vi "Cam0 Ball Target Loop.vi"(0 "Camera Name":string="cam0") -> ()   [LabVIEW 2023]
uses:
  <vilib>/vision/Image Controls.llb/IMAQ Image.ctl
  Camera Set Up/Event Setup Types.ctl
  <vilib>/Rock Robotics/Network Tables/NT Write Numeric Array.vi
  <vilib>/Utility/config.llb/Write Key (String).vi
  <vilib>/Utility/config.llb/Read Key (String).vi
  <vilib>/Utility/config.llb/NI_LVConfig.lvlib
  <vilib>/vision/NI_Vision_Development_Module.lvlib
panel:
  in  "Main":enum32{"Page 1", "Page 2"}(tab)
  out "Algae Distance":dbl[](array[numeric]) caption="Distance" format="%.1f"
  out "Algae Angle":dbl[](array[numeric]) caption="Angle" format="%.1f"
  out "Image":T1(plugin-control)
  in  "Settings":bool
  in  "Save":bool
  in  "Tools":bool
  in  "Home":bool
  out "Ball Fps":dbl format="%#.0f"
  in  "Ball Diameter (in)":dbl=16.0
  in  "FOV":dbl=68.5
  in  "Algae Color Range":T2={"Hue"={21.620689392089844, 69.62068939208984}, "Sat"={66.41378784179688, 255.0}, "Val"={96.0, 255.0}} caption="Color Range" {"Hue" scale=0.0..255.0 scale format="%#_3g"}
  out "Mask":T1(plugin-control)
  in  "Score Threshold %":dbl=80.0
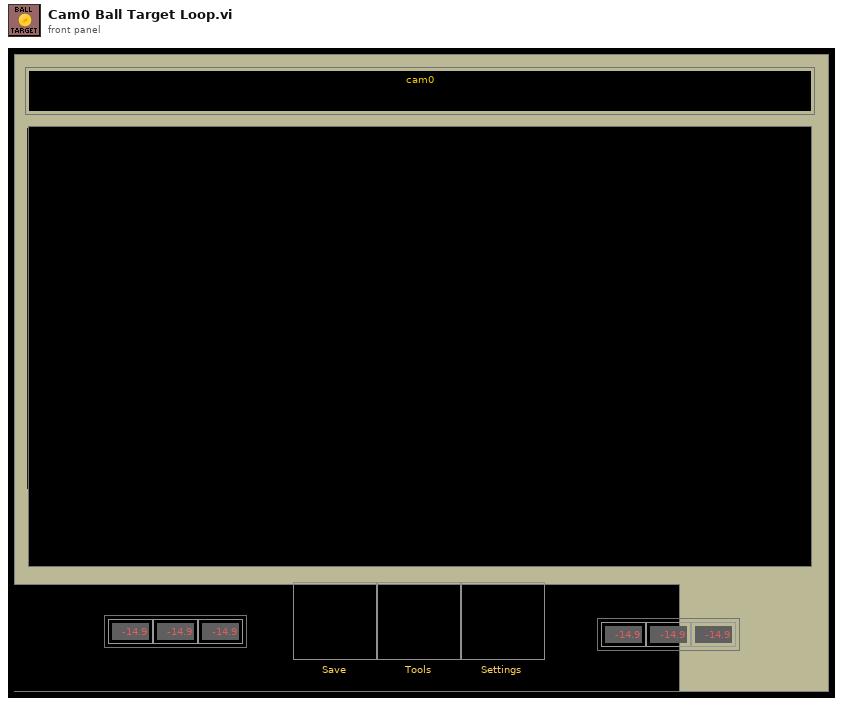
[diagram p1: front panel]
types:
  T1 = typedef "IMAQ Image.ctl" = refnum<image>
  T2 = cluster{"Hue":cluster{dbl, dbl}, "Sat":cluster{dbl, dbl}, "Val":cluster{dbl, dbl}}
  T3 = typedef "Particle Parameters" = i32
  T4 = typedef "Image Type" = u32
  T5 = typedef "Event Setup Types.ctl" = enum16{"Default", "Camera Loop Started", "Save Data", "Open Front Panel", "Exit"}
  T6 = typedef "Target Fields.ctl" = cluster{"diameter points":cluster{"first point":cluster{"x":dbl, "y":dbl}, "projected point":cluster{"x":dbl, "y":dbl}}, "normalized center":cluster{"x":dbl, "y":dbl}, "Overall Score":dbl, "Area Score":dbl, "Moment Score":dbl, "Aspect Score":dbl, "Distance (ft)":dbl, "Upper Goal":bool}
  T7 = typedef "NI_LVConfig.lvlib/Config Data RefNum.ctl" = refnum<k1>
  T8 = cluster{cluster{"Lower":dbl, "Upper":dbl}, cluster{"Lower":dbl, "Upper":dbl}, cluster{"Lower":dbl, "Upper":dbl}}
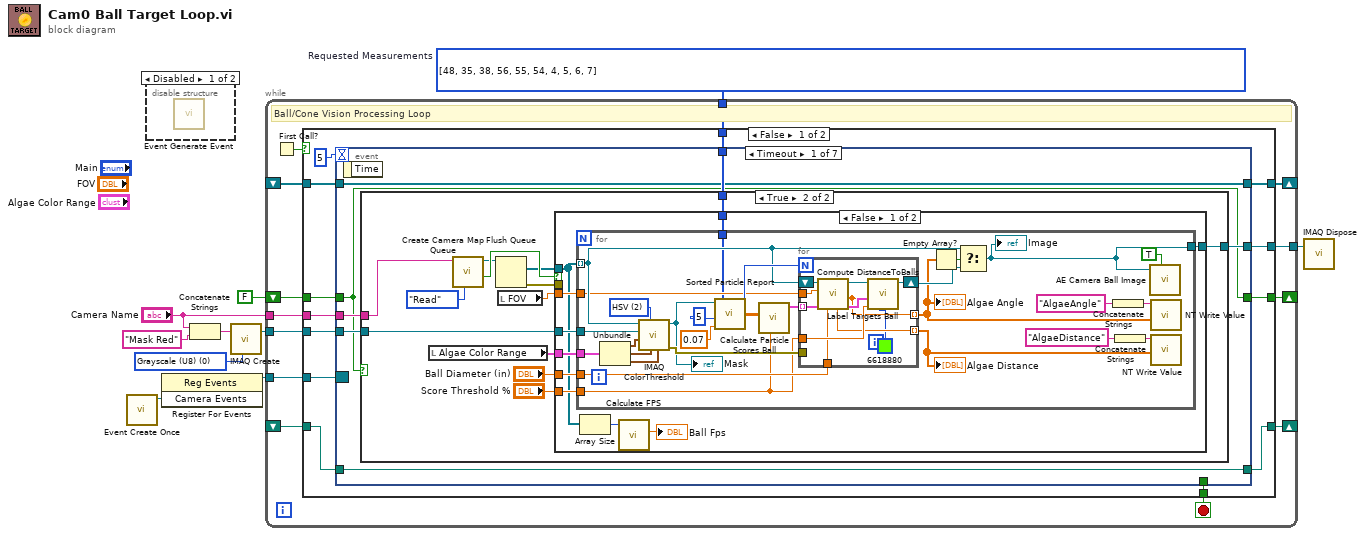
[diagram p0: block diagram]
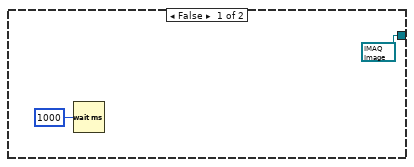
[diagram p3: hidden frame]
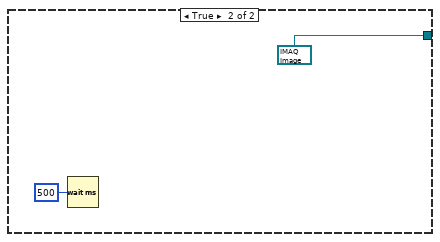
[diagram p4: hidden frame]
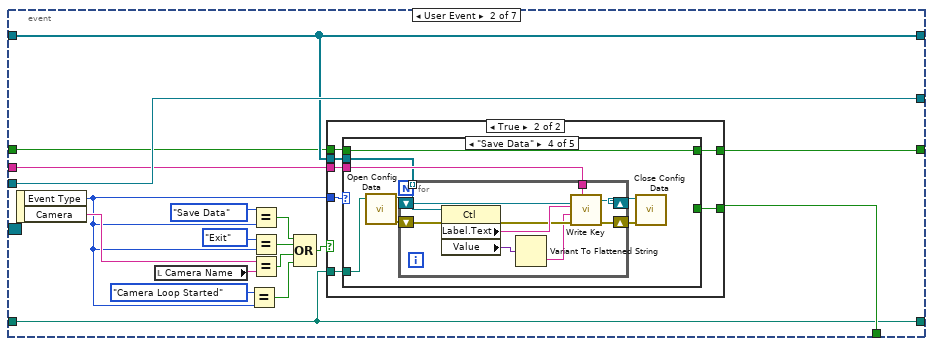
[diagram p5: hidden frame]
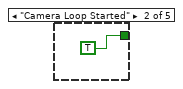
[diagram p8: hidden frame]
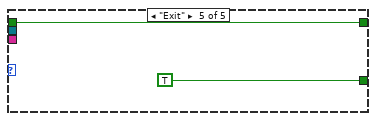
[diagram p10: hidden frame]
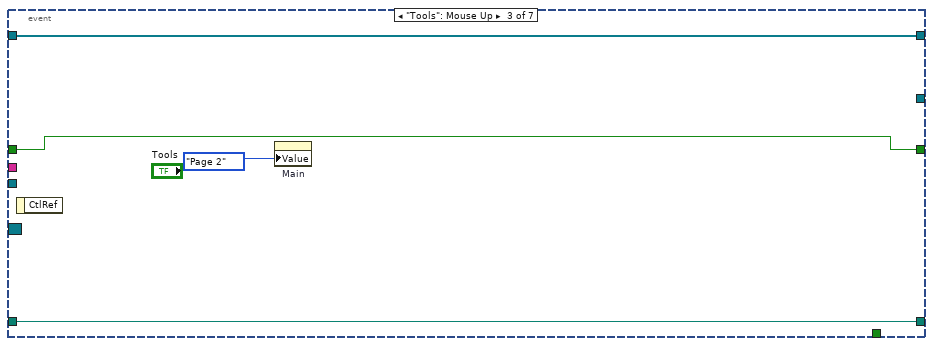
[diagram p11: hidden frame]
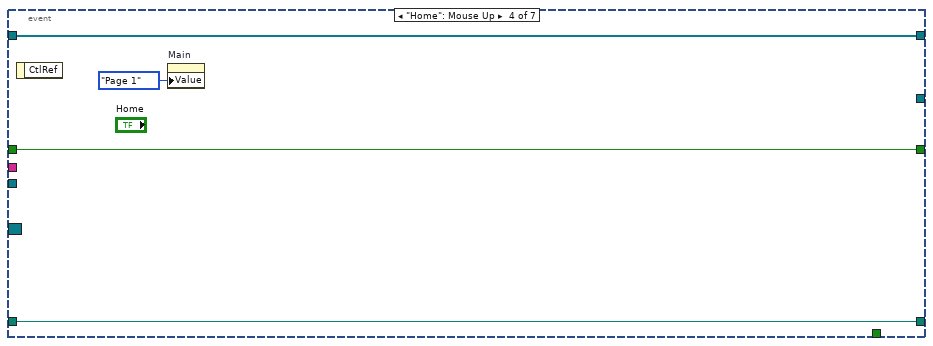
[diagram p12: hidden frame]
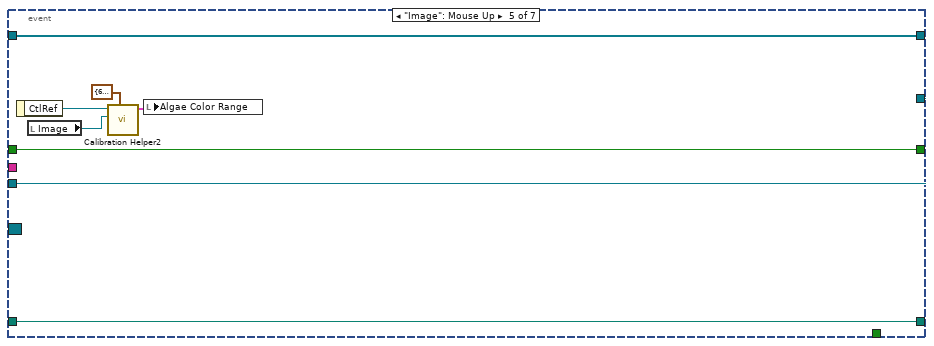
[diagram p13: hidden frame]
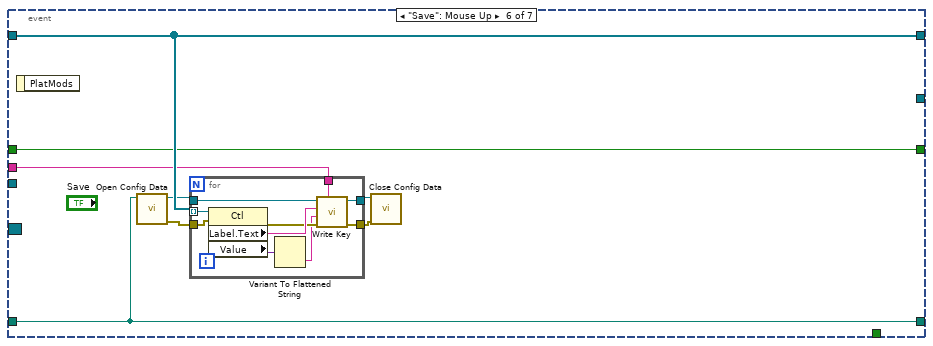
[diagram p14: hidden frame]
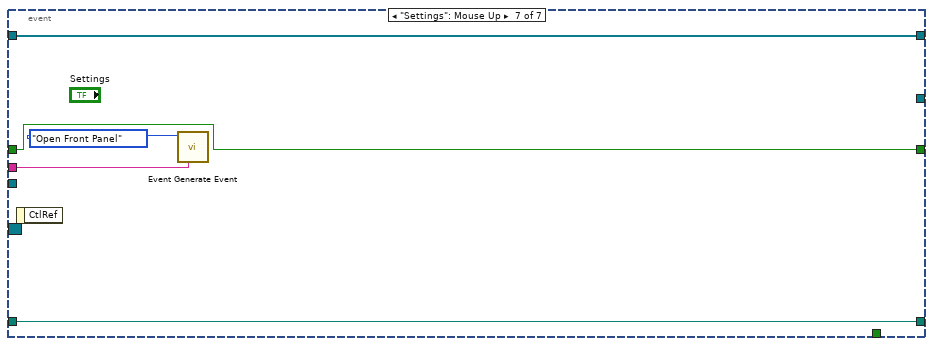
[diagram p15: hidden frame]
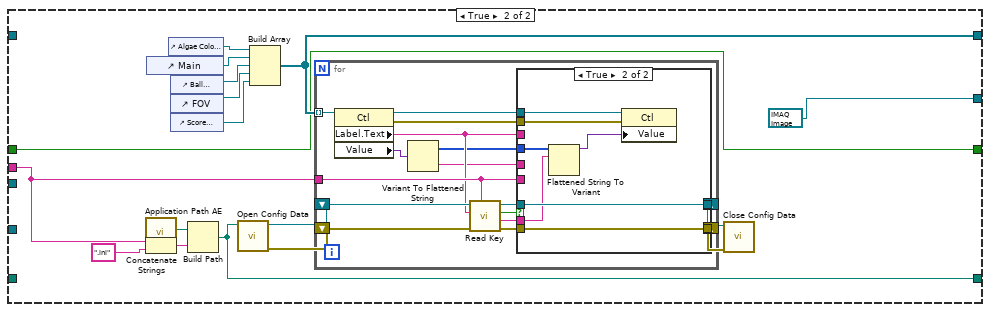
[diagram p16: hidden frame]
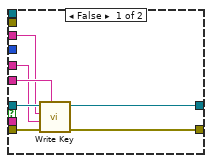
[diagram p17: hidden frame]
diagram:
  w5 = T3[] [48, 35, 38, 56, 55, 54, 4, 5, 6, 7] items=["Center of Mass X", "Center of Mass Y", "First Pixel X", "First Pixel Y", "Bounding Rect Left", "Bounding Rect Top", "Bounding Rect Right", "Bounding Rect Bottom", "Max Feret Diameter Start X", "Max Feret Diameter Start Y", "Max Feret Diameter End X", "Max Feret Diameter End Y", "Max Horiz. Segment Length Left", "Max Horiz. Segment Length Right", "Max Horiz. Segment Length Row", "-", "Bounding Rect Width", "Bounding Rect Height", "Bounding Rect Diagonal", "Perimeter", "Convex Hull Perimeter", "Holes' Perimeter", "Max Feret Diameter", "Equivalent Ellipse Major Axis", "Equivalent Ellipse Minor Axis", "Equivalent Ellipse Minor Axis (Feret)", "Equivalent Rect Long Side", "Equivalent Rect Short Side", "Equivalent Rect Diagonal", "Equivalent Rect Short Side (Feret)", "Average Horiz. Segment Length", "Average Vert. Segment Length", "Hydraulic Radius", "Waddel Disk Diameter", "-", "Area", "Holes' Area", "Particle & Holes' Area", "Convex Hull Area", "Image Area", "-", "Number of Holes", "Number of Horiz. Segments", "Number of Vert. Segments", "-", "Orientation", "Max Feret Diameter Orientation", "-", "% Area/Image Area", "% Area/(Particle & Holes' Area)", "Ratio of Equivalent Ellipse Axes", "Ratio of Equivalent Rect Sides", "-", "Elongation Factor", "Compactness Factor", "Heywood Circularity Factor", "Type Factor", "-", "Sum X", "Sum Y", "Sum XX", "Sum XY", "Sum YY", "Sum XXX", "Sum XXY", "Sum XYY", "Sum YYY", "-", "Moment of Inertia XX", "Moment of Inertia XY", "Moment of Inertia YY", "Moment of Inertia XXX", "Moment of Inertia XXY", "Moment of Inertia XYY", "Moment of Inertia YYY", "Norm. Moment of Inertia XX", "Norm. Moment of Inertia XY", "Norm. Moment of Inertia YY", "Norm. Moment of Inertia XXX", "Norm. Moment of Inertia XXY", "Norm. Moment of Inertia XYY", "Norm. Moment of Inertia YYY", "Hu Moment 1", "Hu Moment 2", "Hu Moment 3", "Hu Moment 4", "Hu Moment 5", "Hu Moment 6", "Hu Moment 7"]  # Requested Measurements
  w6 = T4 0 items=["Grayscale (U8)", "Grayscale (I16)", "Grayscale (SGL)", "Complex (CSG)", "RGB (U32)", "HSL (U32)", "RGB (U64)", "Grayscale (U16)"] ("Image Type")
  n1 = call "Event Create Once.vi"() -> ("Camera Events"=w8:refnum<user-event>)  [unwired: 10 in, 1 out]
  n2 = disable-structure shown="Disabled" {
    frame Disabled {
      n3 = call "Event Generate Event.vi"() -> ()  [unwired: 12 in]
    }
    frame Enabled {
    }
  }
  n4 = register-events(w8) -> (reference out=w7:refnum<event-registration>)  [unwired: 2 in, 1 out]
  n5 = Concatenate Strings("Camera Name", "Mask Red" ("string")) -> (w4:string)
  n6 = call "IMAQ Create"("Image Name"=w4, "Image Type"=w6) -> ("New Image"=w10:T1)  [unwired: 2 in, 2 out]
  n7 = while {
    tunnel: w10 -> [w23]
    tunnel: w5 -> [w22]
    tunnel: [w21] -> w9
    tunnel: w7 -> [w20]
    tunnel: "Camera Name" -> [w18]
    shift-right: [w16] -> _
    shift-left: _ -> [w15]
    shift-right: [w14] -> _
    shift-left: _ -> [w13]
    shift-right: [w11] -> _
    shift-left: FALSE -> [w12]
    stop <- w19 stop-if-true
    # "Ball/Cone Vision Processing Loop"
    n8 = First Call?() -> (First Call?: T/F=w17:bool)
    n9 = case shown="False" w17 {
      tunnel: w23 -> [w36 _]
      tunnel: w22 -> [w35 _]
      tunnel: [w34 T1 refnum ("New Image")] -> w21
      tunnel: w20 -> [w33 _]
      tunnel: [w32 _] -> w19
      tunnel: w18 -> [w31 w208]
      tunnel: [w29 w203] -> w16
      tunnel: w15 -> [w30 _]
      tunnel: [w28 w207] -> w14
      tunnel: w13 -> [w26 _]
      tunnel: w12 -> [w25 w198]
      tunnel: [w24 w198] -> w11
      frame False {
        n10 = event shown="[0] Timeout" {
          selector: w33 -> [_ _ _ _ _ _ _]
          dyn-events: _ -> [_ _ _ _ _ _ _]
          timeout: 5 -> [_ _ _ _ _ _ _]
          tunnel: w36 -> [w41 w127 _ _ w172 _ _]
          tunnel: w35 -> [w43 _ _ _ _ _ _]
          tunnel: [w42 w127 _ _ w172 _ _] -> w34
          tunnel: [_ w126 _ _ _ _ _] -> w32
          tunnel: w31 -> [w38 w125 _ _ _ w178 w194]
          tunnel: w30 -> [w40 w123 w162 w166 w170 w181 w197]
          tunnel: [w40 w123 w162 w166 w170 w181 w197] -> w29
          tunnel: w26 -> [w39 w124 w161 w165 w169 w182 w196]
          tunnel: [w39 w124 w161 w165 w169 w182 w196] -> w28
          tunnel: w25 -> [w37 w114 w159 w163 w167 w175 w193]
          tunnel: [w37 w113 w159 w163 w167 w175 w193] -> w24
          event Timeout {
            n11 = event-data() -> ()  [unwired: 1 in, 1 out]
            n12 = case shown="True" w37 {
              tunnel: w43 -> [_ w58]
              tunnel: [T1 refnum ("Image") w57] -> w42
              tunnel: w41 -> [_ w56]
              tunnel: w38 -> [_ w46]
              frame False {
                n13 = Wait (ms)(milliseconds to wait=u32 1000) -> ()  [unwired: 1 out]
              }
              frame True {
                n14 = local read "Algae Color Range"() -> (w52:T2)
                n15 = call "Create Camera Map Queue.vi"("Action"=enum16{"Read", "Write"}."Read", "Camera"=w46) -> ("key not found?"=w54:bool, "value"=w49:refnum<queue>)  [unwired: 8 in]
                n16 = Flush Queue(queue=w49) -> (remaining elements=w48:T1[], error out=w47:errorcluster)  [unwired: 1 in, 1 out]
                n17 = local read "FOV"() -> (w53:dbl)
                n18 = case shown="False" w54 {
                  tunnel: w58 -> [w68 _]
                  tunnel: [w67 T1 refnum ("Image")] -> w57
                  tunnel: w56 -> [w66 _]
                  tunnel: w53 -> [w65 _]
                  tunnel: w52 -> [w64 _]
                  tunnel: "Ball Diameter (in)" -> [w63 _]
                  tunnel: "Score Threshold %" -> [w62 _]
                  tunnel: w48 -> [w59 _]
                  tunnel: w47 -> [_ _]
                  frame False {
                    n19 = for {
                      tunnel: w66 -> [w91]
                      tunnel: w68 -> [w80]
                      tunnel: w59 -> [w82] mode=indexing
                      tunnel: [w79] -> w67
                      tunnel: w65 -> [w81]
                      tunnel: w64 -> [w86]
                      tunnel: w63 -> [w72]
                      tunnel: w62 -> [w70]
                      w92 = u16 2 items=["RGB", "HSL", "HSV", "HSI"] ("Color Mode")
                      n20 = Unbundle(w86) -> ("Hue"=w85:cluster{dbl, dbl}, "Sat"=w84:cluster{dbl, dbl}, "Val"=w83:cluster{dbl, dbl})
                      n21 = call "IMAQ ColorThreshold"("Blue or Luma or Val or Inten Range"=w83, "Green or Sat Range"=w84, "Color Mode"=w92, "Red or Hue Range"=w85, "Image Dst"=w91, "Image Src"=w82) -> ("error out"=w90:errorcluster, "Image Dst Out"=w71:T1)  [unwired: 4 in]
                      "Mask" <- w71
                      n22 = call "Sorted Particle Report.vi"("Min Area Size %"=0.07 ("Size Limit %"), "Particle Count Limit"=5 ("Particle Count LImit"), "Pixel Measurements"=w80, "Image in"=w71) -> ("Sorted Data"=w95:dbl[][], "Particles"=w89:i32)  [unwired: 1 out]
                      n23 = call "Calculate Particle Scores Ball.vi"("Limit"=w70, "Sorted Data"=w95) -> ("Scores"=w94:T6[])  [unwired: 9 in]
                      n24 = for {
                        N: w89 -> [_]
                        tunnel: w94 -> [w105] mode=indexing
                        shift-right: [w107] -> w88
                        shift-left: w82 -> [w103]
                        tunnel: w70 -> [w106]
                        tunnel: [w100] -> w74 mode=indexing
                        tunnel: w90 -> [_]
                        tunnel: w81 -> [w101]
                        tunnel: [w99] -> w73 mode=indexing
                        tunnel: w72 -> [w97]
                        n25 = call "Compute DistanceToBalls.vi"("Target Width (in)"=w97, "results"=w105, "FOV"=w101, "Image Src"=w103) -> ("results out"=w102:T6, "Off Angle"=w100:dbl, "Image Dst Out"=w104:T1, "Distance"=w99:dbl)  [unwired: 3 in, 1 out]
                        n26 = call "Label Targets Ball.vi"("Color"=u32 6618880, "Score Threshold"=w106, "results"=w102, "Angle"=w100, "Image in"=w104) -> ("Image out"=w107:T1)  [unwired: 6 in]
                      }
                      "Algae Angle" <- w74
                      "Algae Distance" <- w73
                      n27 = Empty Array?(array=w74) -> (empty?=w87:bool)
                      n28 = Select(t=w82, s=w87, f=w88) -> (s? t:f=w79:T1)
                      "Image" <- w79
                      n29 = Concatenate Strings("AlgaeAngle" ("Name")) -> (w75:string)
                      n30 = Concatenate Strings("AlgaeDistance" ("Name")) -> (w76:string)
                      n31 = call "AE Camera Ball Image.vi"("Update"=TRUE, "Ball Image in"=w79) -> ()  [unwired: 9 in, 1 out]
                      n32 = call-poly <vilib>:"NT Write Value.vi"("value"=w74, "name"=w75) -> ()  [unwired: 9 in, 1 out]
                      n33 = call-poly <vilib>:"NT Write Value.vi"("value"=w73, "name"=w76) -> ()  [unwired: 9 in, 1 out]
                    }
                    n34 = Array Size(array=w59) -> (size(s)=w61:i32)
                    n35 = call "Calculate FPS.vi"("Frames Processed"=w61) -> ("Fps"=→"Ball Fps":dbl)  [unwired: 10 in]
                  }
                  frame True {
                    n36 = Wait (ms)(milliseconds to wait=u32 500) -> ()  [unwired: 1 out]
                  }
                }
              }
            }
          }
          event User Event {
            n37 = event-data() -> ("Event Type"=w112:T5, "Camera"=w117:string)  [unwired: 1 in]
            n38 = local read "Camera Name"() -> (w118:string)
            n39 = Equal?(x=Event_Setup_Types."Camera Loop Started", y=w112) -> (x = y?=w110:bool)
            n40 = Equal?(x=Event_Setup_Types."Save Data", y=w112) -> (x = y?=w119:bool)
            n41 = Equal?(x=Event_Setup_Types."Exit", y=w112) -> (x = y?=w121:bool)
            n42 = Equal?(x=w117, y=w118) -> (x = y?=w116:bool)
            n43 = Compound Arithmetic op=OR(w119, w121, w116, w110) -> (w115:bool)
            n44 = case shown="True" w115 {
              tunnel: w112 -> [_ w135]
              tunnel: [_ w134] -> w126
              tunnel: w125 -> [_ w133]
              tunnel: w124 -> [_ w132]
              tunnel: w123 -> [_ w131]
              tunnel: w114 -> [w128 w130]
              tunnel: [w128 w129] -> w113
              frame False {
              }
              frame True {
                n45 = case shown="\"Save Data\"" w135 {
                  tunnel: [_ _ _ _ TRUE] -> w134
                  tunnel: w133 -> [_ _ _ w142 _]
                  tunnel: w132 -> [_ _ _ w141 _]
                  tunnel: w131 -> [_ _ _ w140 _]
                  tunnel: w130 -> [w136 _ w138 w139 w157]
                  tunnel: [w136 TRUE w138 w139 w157] -> w129
                  frame "Default" {
                  }
                  frame "Camera Loop Started" {
                  }
                  frame "Open Front Panel" {
                  }
                  frame "Save Data" {
                    n46 = call <vilib>:"Open Config Data.vi"("configuration file path"=w141) -> ("error out"=w143:errorcluster, "refnum"=w146:T7)  [unwired: 8 in, 1 out]
                    n47 = for {
                      tunnel: w142 -> [w152]
                      tunnel: w140 -> [w151] mode=indexing
                      shift-right: [w155] -> w145
                      shift-left: w146 -> [w156]
                      shift-right: [w154] -> w144
                      shift-left: w143 -> [w153]
                      n48 = property class="Ctl"(reference=w151, error in=w153) -> (error out=w148:errorcluster, "Label.Text"=w150:string, "Value"=w149:variant)  [unwired: 1 out]
                      n49 = Variant To Flattened String(Variant=w149) -> (data string=w147:string)  [unwired: 1 out]
                      n50 = call-poly <vilib>:"Write Key.vi"("section"=w152, "error in (no error)"=w148, "value"=w147, "key"=w150, "refnum"=w156) -> ("error out"=w154:errorcluster, "refnum out"=w155:T7)  [unwired: 4 in, 1 out]
                    }
                    n51 = call <vilib>:"Close Config Data.vi"("error in (no error)"=w144, "refnum"=w145) -> ()  [unwired: 8 in, 2 out]
                  }
                  frame "Exit" {
                  }
                }
              }
            }
          }
          event "Tools": Mouse Up {
            n52 = event-data() -> ()  [unwired: 1 in, 1 out]
            n53 = property on="Main" class="TabCtl (strict)"("Value"=enum32{"Page 1", "Page 2"}."Page 2" ("Main")) -> ()  [unwired: 2 in, 2 out]
          }
          event "Home": Mouse Up {
            n54 = event-data() -> ()  [unwired: 1 in, 1 out]
            n55 = property on="Main" class="TabCtl (strict)"("Value"=enum32{"Page 1", "Page 2"}."Page 1" ("Main")) -> ()  [unwired: 2 in, 2 out]
          }
          event "Image": Mouse Up {
            n56 = event-data() -> ("CtlRef"=w173:refnum<vi>)  [unwired: 1 in]
            n57 = local read "Image"() -> (w171:T1)
            n58 = call "Calibration Helper2.vi"("Std Devs"=cluster{"H":dbl, "S":dbl, "V":dbl} {"H"=6.0, "S"=6.0, "V"=6.0} ("Std Devs Ball"), "Image"=w171, "Image Ctl Refnum"=w173) -> ("output color"=w168:T8)  [unwired: 7 in, 1 out]
            n59 = local write "Algae Color Range"(w168) -> ()
          }
          event "Save": Mouse Up {
            n60 = event-data() -> ()  [unwired: 1 in, 1 out]
            n61 = call <vilib>:"Open Config Data.vi"("configuration file path"=w182) -> ("error out"=w179:errorcluster, "refnum"=w180:T7)  [unwired: 8 in, 1 out]
            n62 = for {
              tunnel: w181 -> [w192] mode=indexing
              tunnel: w180 -> [w191]
              tunnel: w179 -> [w190]
              tunnel: w178 -> [w186]
              tunnel: [w184] -> w177
              tunnel: [w183] -> w176
              n63 = property class="Ctl"(reference=w192, error in=w190) -> (error out=w187:errorcluster, "Label.Text"=w189:string, "Value"=w188:variant)  [unwired: 1 out]
              n64 = Variant To Flattened String(Variant=w188) -> (data string=w185:string)  [unwired: 1 out]
              n65 = call-poly <vilib>:"Write Key.vi"("section"=w186, "error in (no error)"=w187, "value"=w185, "key"=w189, "refnum"=w191) -> ("error out"=w184:errorcluster, "refnum out"=w183:T7)  [unwired: 4 in, 1 out]
            }
            n66 = call <vilib>:"Close Config Data.vi"("error in (no error)"=w177, "refnum"=w176) -> ()  [unwired: 8 in, 2 out]
          }
          event "Settings": Mouse Up {
            n67 = event-data() -> ()  [unwired: 1 in, 1 out]
            n68 = call "Event Generate Event.vi"("Camera Name"=w194, "Event Type"=Event_Setup_Types."Open Front Panel") -> ()  [unwired: 10 in]
          }
        }
      }
      frame True {
        n69 = call "Application Path AE.vi"() -> ("Application Path out"=w205:path)  [unwired: 11 in]
        n70 = Concatenate Strings(w208, ".ini" ("name or relative path")) -> (w213:string)
        n71 = control-ref of="Main"() -> (w202:refnum<vi>)
        n72 = control-ref of="Algae Color Range"() -> (w204:refnum<vi>)
        n73 = control-ref of="Ball Diameter (in)"() -> (w201:refnum<vi>)
        n74 = control-ref of="FOV"() -> (w200:refnum<vi>)
        n75 = control-ref of="Score Threshold %"() -> (w199:refnum<vi>)
        n76 = Build Path(base path=w205, name or relative path=w213) -> (appended path=w207:path)
        n77 = call <vilib>:"Open Config Data.vi"("configuration file path"=w207) -> ("error out"=w206:errorcluster, "refnum"=w212:T7)  [unwired: 8 in, 1 out]
        n78 = Build Array(w204, w202, w201, w200, w199) -> (w203:refnum<vi>[])
        n79 = for {
          tunnel: w208 -> [w227]
          tunnel: w203 -> [w217] mode=indexing
          shift-right: [w229] -> w211
          shift-left: w212 -> [w230]
          shift-right: [w228] -> w210
          shift-left: w206 -> [w226]
          n80 = property class="Ctl"(reference=w217) -> (reference out=w223:refnum<vi>, error out=w222:errorcluster, "Label.Text"=w220:string, "Value"=w216:variant)  [unwired: 1 in]
          n81 = Variant To Flattened String(Variant=w216) -> (data string=w218:string, 1:w215:i16[])
          n82 = call-poly <vilib>:"Read Key.vi"("section"=w227, "error in (no error)"=w226, "key"=w220, "refnum"=w230) -> ("error out"=w219:errorcluster, "value"=w224:string, "found?"=w225:bool, "refnum out"=w221:T7)  [unwired: 4 in]
          n83 = case shown="True" w225 {
            tunnel: w224 -> [_ w239]
            tunnel: w223 -> [_ w244]
            tunnel: w222 -> [_ w243]
            tunnel: w221 -> [w237 w242]
            tunnel: w227 -> [w236 _]
            tunnel: w220 -> [w235 _]
            tunnel: [w234 w242] -> w229
            tunnel: w219 -> [w233 w241]
            tunnel: [w232 w241] -> w228
            tunnel: w218 -> [w231 _]
            tunnel: w215 -> [_ w238]
            frame False {
              n84 = call-poly <vilib>:"Write Key.vi"("section"=w236, "error in (no error)"=w233, "value"=w231, "key"=w235, "refnum"=w237) -> ("error out"=w232:errorcluster, "refnum out"=w234:T7)  [unwired: 4 in, 1 out]
            }
            frame True {
              n85 = Flattened String To Variant(6:w239, 7:w238) -> (3:w240:variant)  [unwired: 1 in, 1 out]
              n86 = property class="Ctl"(reference=w244, error in=w243, "Value"=w240) -> ()  [unwired: 2 out]
            }
          }
        }
        n87 = call <vilib>:"Close Config Data.vi"("error in (no error)"=w210, "refnum"=w211) -> ()  [unwired: 8 in, 2 out]
      }
    }
  }
  n88 = call "IMAQ Dispose"("Image"=w9) -> ()  [unwired: 5 in, 1 out]
